vi "GetSelectionList.vi"(8 "error in (no error)":errorcluster caption="错误输入（无错误）", 11 "XYPlot 输入":refnum<class "XYPlot.lvclass">) -> (0 "error out":errorcluster caption="错误输出", 3 "XYPlot 输出":refnum<class "XYPlot.lvclass">)   [LabVIEW 2018, in "DataDisplay.lvlib" / "XYPlot.lvclass"]
uses:
  XYPlot.lvclass
  XYPlot.lvclass/XYPlot.ctl
  SubVI/DD_Parameter.vi
  DataDisplay.lvlib
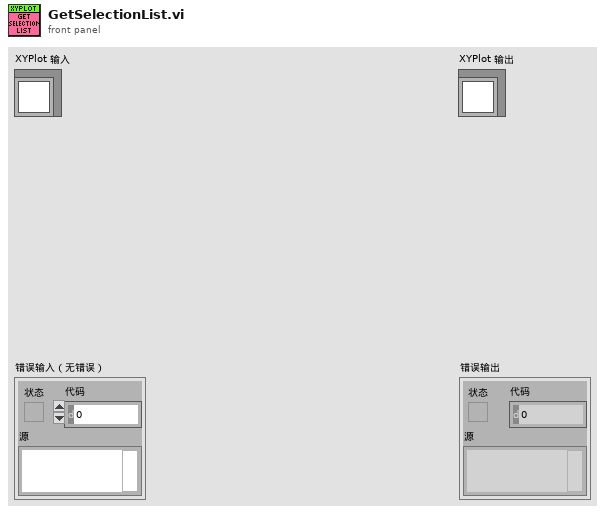
[diagram p1: front panel]
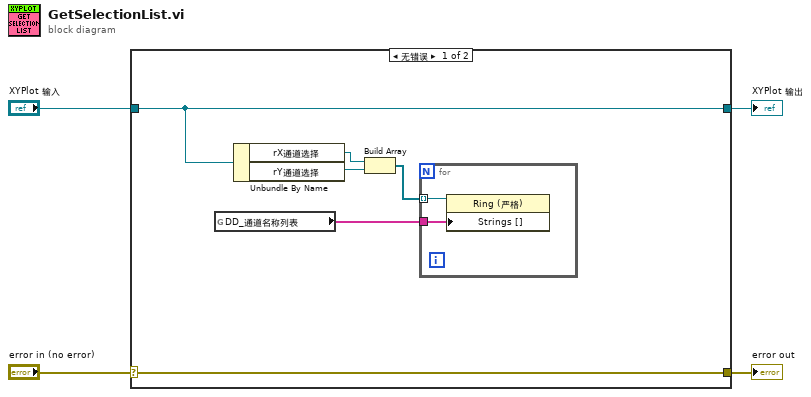
[diagram p0: block diagram]
diagram:
  n1 = case shown="无错误" "error in (no error)" {
    selector: "error in (no error)" -> [w10 w14]
    tunnel: [w10 w14] -> w3
    tunnel: [w9 w13] -> w1
    tunnel: "XYPlot 输入" -> [w9 w13]
    frame No Error {
      n2 = global read "DD_Parameter.vi" "DD_通道名称列表"() -> (w5:string[])
      n3 = Unbundle By Name(w9) -> ("rX通道选择"=w8:refnum<vi>, "rY通道选择"=w7:refnum<vi>)
      n4 = Build Array(w8, w7) -> (w6:refnum<vi>[])
      n5 = for {
        tunnel: w6 -> [w12] mode=indexing
        tunnel: w5 -> [w11]
        n6 = property class="Ring (严格)"(reference=w12, "Strings []"=w11) -> ()  [unwired: 1 in, 2 out]
      }
    }
    frame Error {
    }
  }
  "error out" <- w3
  "XYPlot 输出" <- w1
